vi "Make Channels Coincident Low.vi"(8 "interp. method":i32(ring) items=["nearest", "linear", "spline", "cubic Hermite", "Lagrange"], 9 "Cluster 2":T1={"Colour"=0, "Inst type"=enum."Pitot-static tube", "Inst name"="Manometer voltage", "Symbol"="U", "Code name"="", "Extra Info"="U", "Inst Array"=enum."PWA", "Index"=0, "Voltage Index"=0, "Extra Titles"=[], "Extra Values"=[], "Eng Values"=[], "Time (ms)"=[], "TT / Voltage"=[], "U"=0.0, "u^2"=0.0, "u^3"=0.0, "u^4"=0.0, "Skew_u"=0.0, "Kurt_u"=0.0, "Mean % Err"=0.0, "% u'/U"=0.0} {"Skew_u" format="%.2f"; "% u'/U" format="%.2f"; "Mean % Err" format="%.2f"; "Kurt_u" format="%.2f"; "u^4" format="%.2f"; "u^3" format="%.2f"; "U" format="%.2f"; "u^2" format="%.2f"}, 11 "Cluster 1":T1={"Colour"=0, "Inst type"=enum."Pitot-static tube", "Inst name"="Manometer voltage", "Symbol"="U", "Code name"="", "Extra Info"="U", "Inst Array"=enum."PWA", "Index"=0, "Voltage Index"=0, "Extra Titles"=[], "Extra Values"=[], "Eng Values"=[], "Time (ms)"=[], "TT / Voltage"=[], "U"=0.0, "u^2"=0.0, "u^3"=0.0, "u^4"=0.0, "Skew_u"=0.0, "Kurt_u"=0.0, "Mean % Err"=0.0, "% u'/U"=0.0} {"Skew_u" format="%.2f"; "% u'/U" format="%.2f"; "Mean % Err" format="%.2f"; "Kurt_u" format="%.2f"; "u^4" format="%.2f"; "u^3" format="%.2f"; "U" format="%.2f"; "u^2" format="%.2f"}) -> (1 "Coincident Channel 2":T1={"Colour"=0, "Inst type"=enum."Pitot-static tube", "Inst name"="Manometer voltage", "Symbol"="U", "Code name"="", "Extra Info"="U", "Inst Array"=enum."PWA", "Index"=0, "Voltage Index"=0, "Extra Titles"=[], "Extra Values"=[], "Eng Values"=[], "Time (ms)"=[], "TT / Voltage"=[], "U"=0.0, "u^2"=0.0, "u^3"=0.0, "u^4"=0.0, "Skew_u"=0.0, "Kurt_u"=0.0, "Mean % Err"=0.0, "% u'/U"=0.0} {"Skew_u" format="%.2f"; "% u'/U" format="%.2f"; "Mean % Err" format="%.2f"; "Kurt_u" format="%.2f"; "u^4" format="%.2f"; "u^3" format="%.2f"; "U" format="%.2f"; "u^2" format="%.2f"}, 3 "Coincident Channel 1":T1={"Colour"=0, "Inst type"=enum."Pitot-static tube", "Inst name"="Manometer voltage", "Symbol"="U", "Code name"="", "Extra Info"="U", "Inst Array"=enum."PWA", "Index"=0, "Voltage Index"=0, "Extra Titles"=[], "Extra Values"=[], "Eng Values"=[], "Time (ms)"=[], "TT / Voltage"=[], "U"=0.0, "u^2"=0.0, "u^3"=0.0, "u^4"=0.0, "Skew_u"=0.0, "Kurt_u"=0.0, "Mean % Err"=0.0, "% u'/U"=0.0} {"Skew_u" format="%.2f"; "% u'/U" format="%.2f"; "Mean % Err" format="%.2f"; "Kurt_u" format="%.2f"; "u^4" format="%.2f"; "u^3" format="%.2f"; "U" format="%.2f"; "u^2" format="%.2f"})   [LabVIEW 2011]
uses:
  Controls/Analysis_info_cluster.ctl
  Controls/Inst_type.ctl
  Controls/Instrument_Array.ctl
  <vilib>/gmath/NI_Gmath.lvlib
panel:
  out "Ref size":i32
  out "Interp size":i32
  out "T1 and T2 made coincident 2":cluster{"yi":dbl[], "yi":dbl[]}[](graph)
  out "U1 and U2 made coincident":cluster{"yi":dbl[], "yi":dbl[]}[](graph)
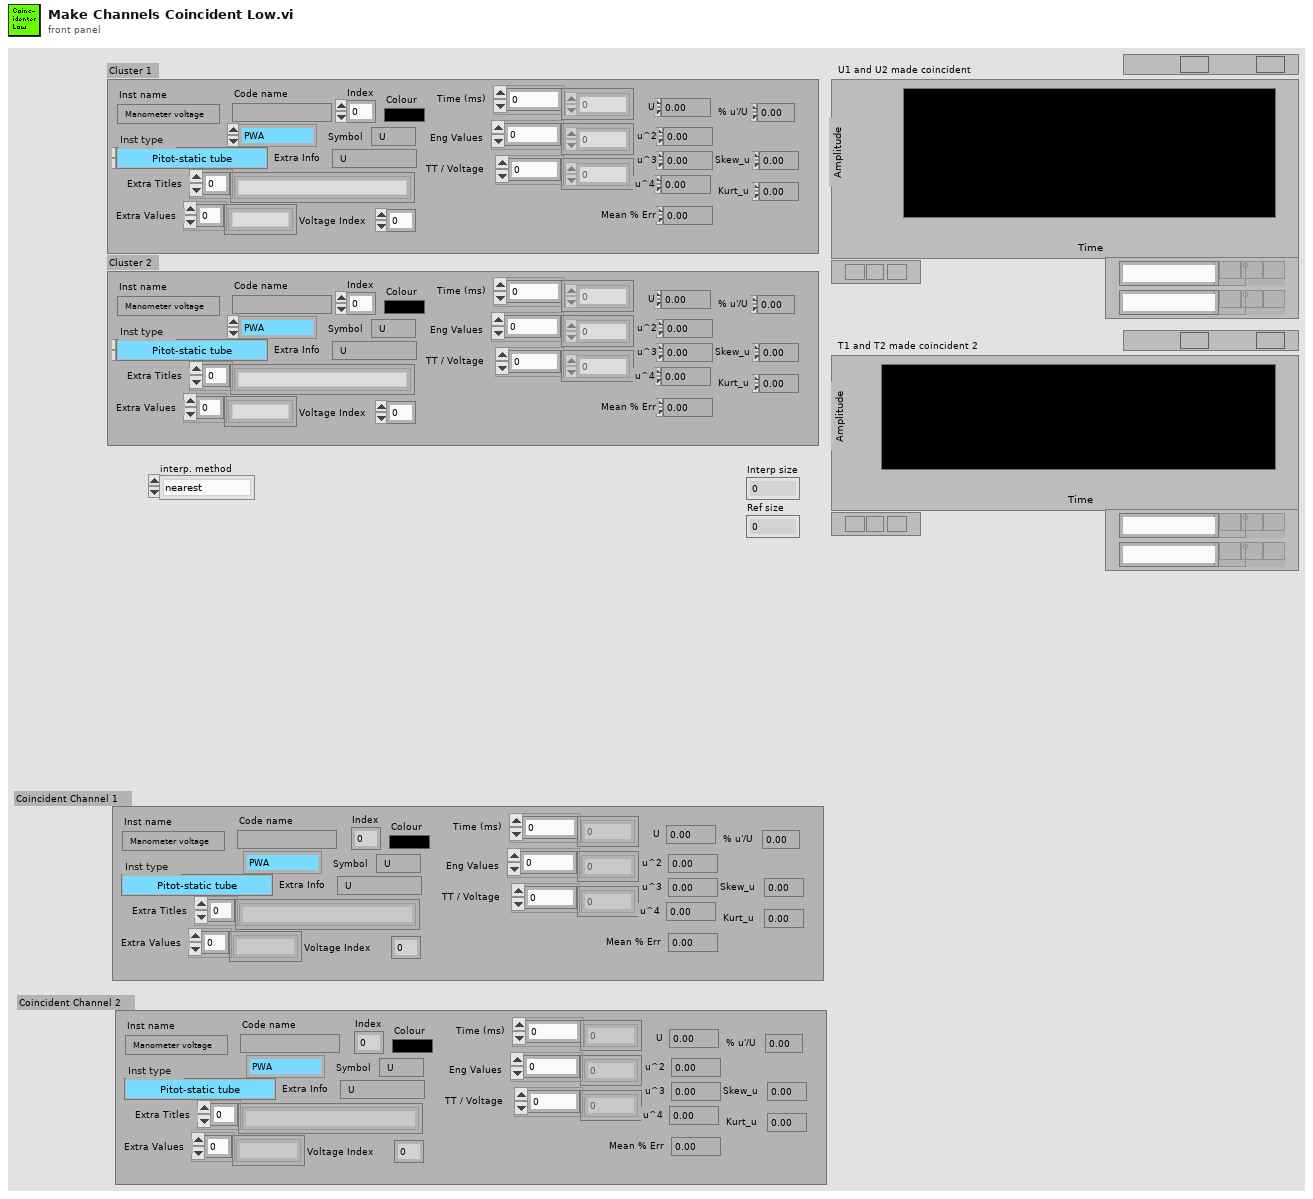
[diagram p1: front panel]
types:
  T1 = typedef "Analysis_info_cluster.ctl" = cluster{"Colour":u32, "Inst type":T2, "Inst name":string, "Symbol":string, "Code name":string, "Extra Info":string, "Inst Array":T3, "Index":i32, "Voltage Index":i32, "Extra Titles":string[], "Extra Values":string[], "Eng Values":dbl[], "Time (ms)":dbl[], "TT / Voltage":dbl[], "U":dbl, "u^2":dbl, "u^3":dbl, "u^4":dbl, "Skew_u":dbl, "Kurt_u":dbl, "Mean % Err":dbl, "% u'/U":dbl}
  T2 = typedef "Inst_type.ctl" = enum16{"Propeller anemometer", "Raw voltage", "Pressure Transducer", "Pitot-static tube", "Preston tube", "Hot wire", "Cross wire 1", "Cross wire 2", "Generic Linear", "Generic Polynomial", "Generic BackPoly", "Fast FID", "Thermocouple", "Cold wire", "Pulsed Wire", "LDA Vel", "LDA Tran time", "LDA Arr time"}
  T3 = typedef "Instrument_Array.ctl" = enum16{"PWA", "LDA", "Analogue"}
  T4 = cluster{"Time (ms)":dbl[], "Eng Values":dbl[], "TT / Voltage":dbl[]}
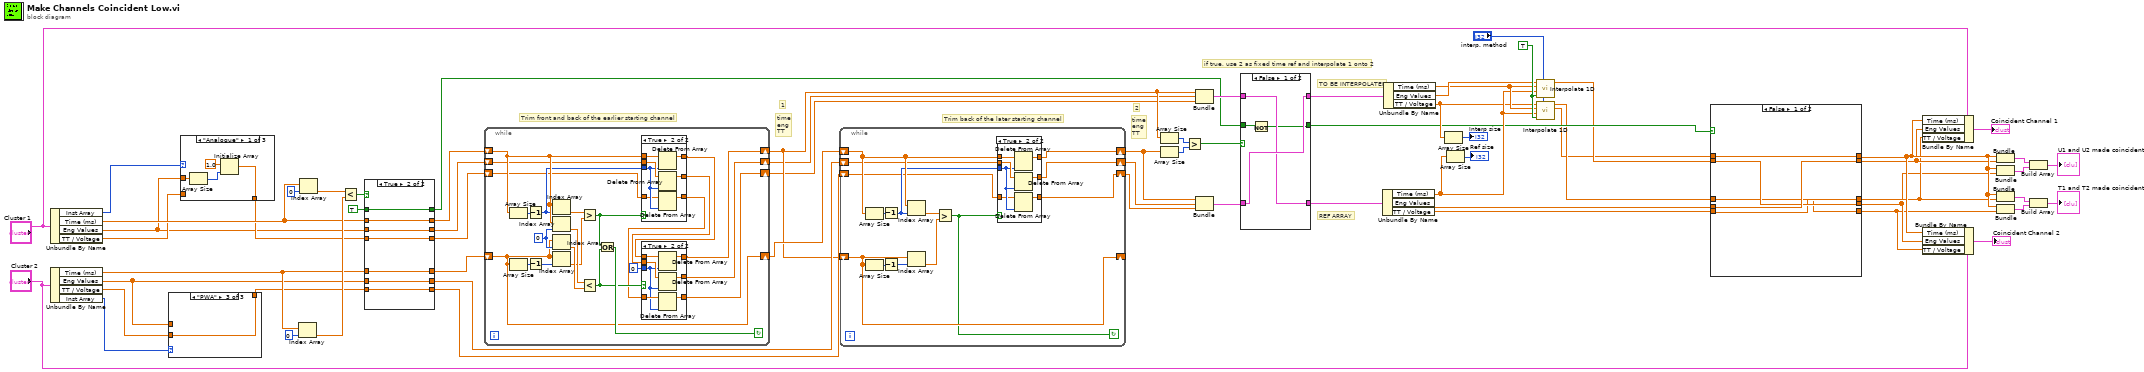
[diagram p0: block diagram]
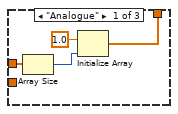
[diagram p2: hidden frame]
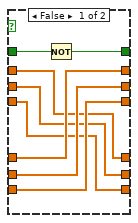
[diagram p9: hidden frame]
diagram:
  w39 = TRUE ("X is monotonic")
  # "Trim back of the later starting channel"
  # "Trim front and back of the earlier starting channel"
  # "TO BE INTERPOLATED"
  # "REF ARRAY"
  # "if true, use 2 as fixed time ref and interpolate 1 onto 2"
  # "2"
  # "1"
  # "time\neng\nTT"
  # "time\neng\nTT"
  n1 = Unbundle By Name("Cluster 1") -> ("Inst Array"=w5:T3, "Time (ms)"=w61:dbl[], "Eng Values"=w16:dbl[], "TT / Voltage"=w17:dbl[])
  n2 = Unbundle By Name("Cluster 2") -> ("Time (ms)"=w56:dbl[], "Eng Values"=w1:dbl[], "TT / Voltage"=w4:dbl[], "Inst Array"=w3:T3)
  n3 = case shown="\"PWA\"" w3 {
    tunnel: w4 -> [_ w71 w72]
    tunnel: [w68 w71 w72] -> w2
    tunnel: w1 -> [w67 _ _]
    frame "Analogue" {
      n4 = Array Size(array=w67) -> (size(s)=w69:i32)
      n5 = Initialize Array(1.0 ("element"), w69) -> (w68:dbl[])
    }
    frame "LDA" {
    }
    frame "PWA" {
    }
  }
  n6 = case shown="\"Analogue\"" w5 {
    tunnel: [w73 w77 w78] -> w18
    tunnel: w17 -> [_ w77 w78]
    tunnel: w16 -> [w75 _ _]
    frame "Analogue" {
      n7 = Array Size(array=w75) -> (size(s)=w74:i32)
      n8 = Initialize Array(1.0 ("element"), w74) -> (w73:dbl[])
    }
    frame "LDA" {
    }
    frame "PWA" {
    }
  }
  n9 = Index Array(array=w56, index=0) -> (element=w63:dbl)
  n10 = Index Array(array=w61, index=0) -> (element=w64:dbl)
  n11 = Less?(x=w64, y=w63) -> (x < y?=w62:bool)
  n12 = case shown="True" w62 {
    tunnel: w61 -> [w81 w93]
    tunnel: [w86 w93] -> w60
    tunnel: [w85 w92] -> w59
    tunnel: w16 -> [w82 w92]
    tunnel: [w84 w91] -> w58
    tunnel: w18 -> [w83 w91]
    tunnel: [w81 w90] -> w57
    tunnel: w56 -> [w86 w90]
    tunnel: [w82 w89] -> w54
    tunnel: w1 -> [w85 w89]
    tunnel: [w83 w88] -> w53
    tunnel: w2 -> [w84 w88]
    tunnel: TRUE -> [w80 w87]
    tunnel: [w79 w87] -> w20
    frame False {
      n13 = Not(x=w80) -> (.not. x?=w79:bool)
    }
    frame True {
    }
  }
  n14 = while {
    shift-right: [w104] -> w47
    shift-left: w60 -> [w109]
    shift-right: [w103] -> w46
    shift-left: w59 -> [w108]
    shift-right: [w94] -> w55
    shift-left: w57 -> [w94]
    shift-right: [w95] -> w45
    shift-left: w58 -> [w97]
    stop <- w110 continue-if-true
    w116 = 0 ("index")
    n15 = Array Size(array=w109) -> (size(s)=w101:i32)
    n16 = Array Size(array=w94) -> (size(s)=w99:i32)
    n17 = Decrement(x=w101) -> (x-1=w100:i32)
    n18 = Decrement(x=w99) -> (x-1=w98:i32)
    n19 = Index Array(array=w109, index=w100) -> (element=w113:dbl)
    n20 = Index Array(array=w109, index=w116) -> (element=w115:dbl)
    n21 = Index Array(array=w94, index=w116) -> (element=w114:dbl)
    n22 = Index Array(array=w94, index=w98) -> (element=w112:dbl)
    n23 = Greater?(x=w113, y=w112) -> (0:w111:bool)
    n24 = Less?(x=w115, y=w114) -> (x < y?=w107:bool)
    n25 = Or(x=w111, y=w107) -> (x .or. y?=w110:bool)
    n26 = case shown="True" w111 {
      tunnel: w109 -> [w129 w135]
      tunnel: w108 -> [w128 w136]
      tunnel: w100 -> [_ w132]
      tunnel: [w129 w134] -> w106
      tunnel: [w128 w133] -> w105
      tunnel: [w127 w131] -> w96
      tunnel: w97 -> [w127 w130]
      frame False {
      }
      frame True {
        n27 = Delete From Array(array=w135, index=w132) -> (array with subset deleted=w134:dbl[])  [unwired: 1 in, 1 out]
        n28 = Delete From Array(array=w136, index=w132) -> (array with subset deleted=w133:dbl[])  [unwired: 1 in, 1 out]
        n29 = Delete From Array(array=w130, index=w132) -> (array with subset deleted=w131:dbl[])  [unwired: 1 in, 1 out]
      }
    }
    n30 = case shown="True" w107 {
      tunnel: w106 -> [w119 w125]
      tunnel: w105 -> [w118 w126]
      tunnel: 0 -> [_ w120]
      tunnel: [w119 w124] -> w104
      tunnel: [w118 w123] -> w103
      tunnel: w96 -> [w117 w122]
      tunnel: [w117 w121] -> w95
      frame False {
      }
      frame True {
        n31 = Delete From Array(array=w125, index=w120) -> (array with subset deleted=w124:dbl[])  [unwired: 1 in, 1 out]
        n32 = Delete From Array(array=w126, index=w120) -> (array with subset deleted=w123:dbl[])  [unwired: 1 in, 1 out]
        n33 = Delete From Array(array=w122, index=w120) -> (array with subset deleted=w121:dbl[])  [unwired: 1 in, 1 out]
      }
    }
  }
  n34 = while {
    shift-right: [w139] -> w48
    shift-left: w55 -> [w148]
    shift-right: [w138] -> w49
    shift-left: w54 -> [w147]
    shift-right: [w141] -> _
    shift-left: w47 -> [w141]
    shift-right: [w137] -> w50
    shift-left: w53 -> [w142]
    stop <- w140 continue-if-true
    n35 = Array Size(array=w148) -> (size(s)=w146:i32)
    n36 = Array Size(array=w141) -> (size(s)=w144:i32)
    n37 = Decrement(x=w146) -> (x-1=w145:i32)
    n38 = Decrement(x=w144) -> (x-1=w143:i32)
    n39 = Index Array(array=w148, index=w145) -> (element=w150:dbl)
    n40 = Index Array(array=w141, index=w143) -> (element=w149:dbl)
    n41 = Greater?(x=w150, y=w149) -> (0:w140:bool)
    n42 = case shown="True" w140 {
      tunnel: w148 -> [w153 w159]
      tunnel: w147 -> [w152 w160]
      tunnel: w145 -> [_ w156]
      tunnel: [w153 w158] -> w139
      tunnel: [w152 w157] -> w138
      tunnel: [w151 w155] -> w137
      tunnel: w142 -> [w151 w154]
      frame False {
      }
      frame True {
        n43 = Delete From Array(array=w159, index=w156) -> (array with subset deleted=w158:dbl[])  [unwired: 1 in, 1 out]
        n44 = Delete From Array(array=w160, index=w156) -> (array with subset deleted=w157:dbl[])  [unwired: 1 in, 1 out]
        n45 = Delete From Array(array=w154, index=w156) -> (array with subset deleted=w155:dbl[])  [unwired: 1 in, 1 out]
      }
    }
  }
  n46 = Array Size(array=w47) -> (size(s)=w52:i32)
  n47 = Array Size(array=w48) -> (size(s)=w51:i32)
  n48 = Greater?(x=w52, y=w51) -> (0:w27:bool)
  n49 = Bundle("Time (ms)"=w47, "Eng Values"=w46, "TT / Voltage"=w45) -> (w44:T4)  [unwired: 1 in]
  n50 = Bundle("Time (ms)"=w48, "Eng Values"=w49, "TT / Voltage"=w50) -> (w43:T4)  [unwired: 1 in]
  n51 = case shown="False" w27 {
    tunnel: w44 -> [w163 w166]
    tunnel: w43 -> [w164 w167]
    tunnel: [w163 w167] -> w41
    tunnel: [w164 w166] -> w42
    tunnel: [w161 w165] -> w21
    tunnel: w20 -> [w162 w165]
    frame False {
      n52 = Not(x=w162) -> (.not. x?=w161:bool)
    }
    frame True {
    }
  }
  n53 = Unbundle By Name(w41) -> ("Time (ms)"=w31:dbl[], "Eng Values"=w13:dbl[], "TT / Voltage"=w12:dbl[])
  n54 = Unbundle By Name(w42) -> ("Time (ms)"=w34:dbl[], "Eng Values"=w38:dbl[], "TT / Voltage"=w30:dbl[])
  n55 = Array Size(array=w30) -> (size(s)=→"Interp size":i32)
  n56 = Array Size(array=w31) -> (size(s)=→"Ref size":i32)
  n57 = call <vilib>:"Interpolate 1D.vi"("method"="interp. method", "X is monotonic"=w39, "xi"=w31, "X"=w34, "Y"=w38) -> ("yi"=w15:dbl[])  [unwired: 1 in, 5 out]
  n58 = call <vilib>:"Interpolate 1D.vi"("method"="interp. method", "X is monotonic"=w39, "xi"=w31, "X"=w34, "Y"=w30) -> ("xi used"=w11:dbl[], "yi"=w14:dbl[])  [unwired: 1 in, 4 out]
  n59 = case shown="False" w21 {
    tunnel: [w172 w177] -> w10
    tunnel: w11 -> [w172 w177]
    tunnel: [w171 w176] -> w9
    tunnel: w15 -> [w170 w176]
    tunnel: w14 -> [w168 w175]
    tunnel: [w169 w175] -> w8
    tunnel: w13 -> [w171 w174]
    tunnel: [w170 w174] -> w7
    tunnel: [w168 w173] -> w6
    tunnel: w12 -> [w169 w173]
    tunnel: w11 -> [_ _]
    frame False {
    }
    frame True {
    }
  }
  n60 = Bundle By Name(cluster="Cluster 1", "Time (ms)"=w10, "Eng Values"=w9, "TT / Voltage"=w8) -> (→"Coincident Channel 1":T1)
  n61 = Bundle By Name(cluster="Cluster 2", "Time (ms)"=w10, "Eng Values"=w7, "TT / Voltage"=w6) -> (→"Coincident Channel 2":T1)
  n62 = Bundle("xi used"=w10, "yi"=w9) -> (w36:cluster{"xi used":dbl[], "yi":dbl[]})  [unwired: 1 in]
  n63 = Bundle("xi used"=w10, "Eng Values"=w7) -> (w37:cluster{"xi used":dbl[], "Eng Values":dbl[]})  [unwired: 1 in]
  n64 = Bundle("xi used"=w10, "yi"=w8) -> (w26:cluster{"xi used":dbl[], "yi":dbl[]})  [unwired: 1 in]
  n65 = Bundle("xi used"=w10, "TT / Voltage"=w6) -> (w32:cluster{"xi used":dbl[], "TT / Voltage":dbl[]})  [unwired: 1 in]
  n66 = Build Array(w36, w37) -> (→"U1 and U2 made coincident":cluster{"xi used":dbl[], "Eng Values":dbl[]}[])
  n67 = Build Array(w26, w32) -> (→"T1 and T2 made coincident 2":cluster{"xi used":dbl[], "TT / Voltage":dbl[]}[])
